vi "Data Access.vi"(10 "Time Out In ms":i32=-1, 11 "2D U16 Group With ID DVR Queue in":refnum<class "2D U16 Group With ID DVR Queue.lvclass">) -> (0 "Time Out":bool, 2 "Data Out":T1, 3 "2D U16 Group With ID DVR Queue out":refnum<class "2D U16 Group With ID DVR Queue.lvclass">)   [LabVIEW 2024, in "2D U16 Group With ID DVR Queue.lvclass"]
uses:
  2D U16 Group With ID DVR Queue.lvclass
  Type Def/Data Type.ctl
  2D U16 Group With ID DVR Queue.lvclass/2D U16 Group With ID DVR Queue.ctl
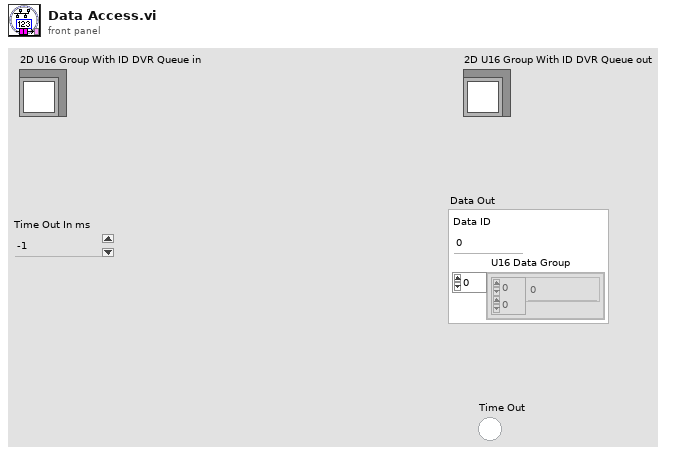
[diagram p1: front panel]
types:
  T1 = typedef "Data Type.ctl" = cluster{"Data ID":i64, "U16 Data Group":cluster{"Array":u16[][]}[]}
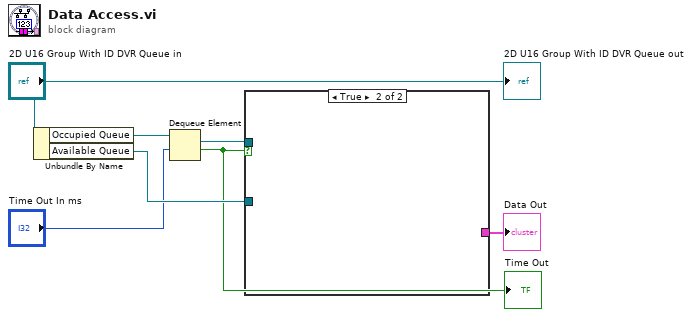
[diagram p0: block diagram]
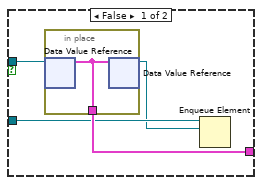
[diagram p2: hidden frame]
diagram:
  n1 = Unbundle By Name("2D U16 Group With ID DVR Queue in") -> ("Occupied Queue"=w5:refnum<queue>, "Available Queue"=w7:refnum<queue>)
  n2 = Dequeue Element(queue=w5, timeout in ms (-1)="Time Out In ms") -> (element=w4:refnum<data-value>, timed out?=w3:bool)  [unwired: 1 in, 2 out]
  "Time Out" <- w3
  n3 = case shown="True" w3 {
    tunnel: [w11 _] -> w1
    tunnel: w4 -> [w9 _]
    tunnel: w7 -> [w10 _]
    frame False {
      n4 = in-place {
        in-place-border: [w12] -> w11
        n5 = in-place-dvr #1(w9) -> (w12:T1)  [unwired: 1 out]
        n6 = in-place-dvr #1(w12) -> (w8:refnum<data-value>)  [unwired: 1 out]
      }
      n7 = Enqueue Element(queue=w10, element=w8) -> ()  [unwired: 2 in, 3 out]
    }
    frame True {
    }
  }
  "Data Out" <- w1
  "2D U16 Group With ID DVR Queue out" <- "2D U16 Group With ID DVR Queue in"
